vi "Check Adept Runtime.vi"(8 "Error In":errorcluster) -> (0 "Error Out":errorcluster, 2 "Installed?":bool)   [LabVIEW 2011]
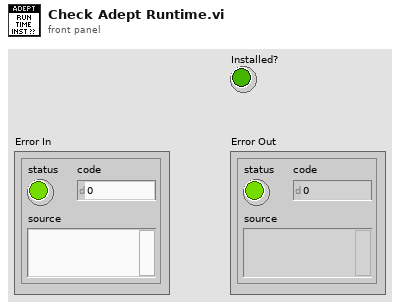
[diagram p1: front panel]
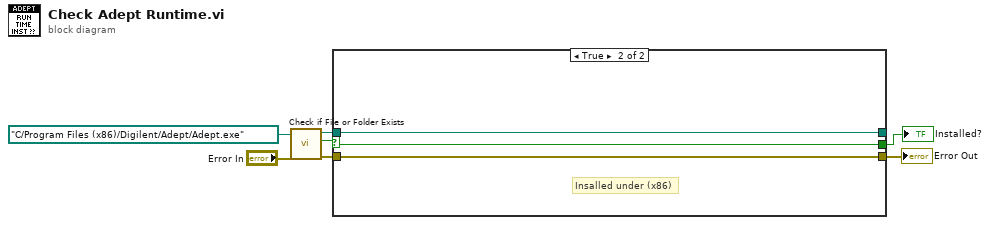
[diagram p0: block diagram]
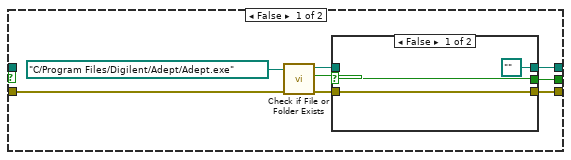
[diagram p2: hidden frame]
diagram:
  n1 = call <vilib>:"Check if File or Folder Exists.vi"("error in (no error)"="Error In", "path"=path "C:/Program Files (x86)/Digilent/Adept/Adept.exe") -> ("error out"=w4:errorcluster, "file or folder exists?"=w6:bool, "dup path"=w5:path)  [unwired: 7 in]
  n2 = case shown="True" w6 {
    selector: w6 -> [_ w22]
    tunnel: w5 -> [_ w24]
    tunnel: w4 -> [w14 w23]
    tunnel: [w13 w24] -> _
    tunnel: [w9 w23] -> w2
    tunnel: [w8 w22] -> w1
    frame False {
      n3 = call <vilib>:"Check if File or Folder Exists.vi"("error in (no error)"=w14, "path"=path "C:/Program Files/Digilent/Adept/Adept.exe") -> ("error out"=w10:errorcluster, "file or folder exists?"=w11:bool, "dup path"=w12:path)  [unwired: 7 in]
      n4 = case shown="False" w11 {
        selector: w11 -> [w17 w19]
        tunnel: [path "" ("dup path") w21] -> w13
        tunnel: w12 -> [_ w21]
        tunnel: w10 -> [w18 w20]
        tunnel: [w18 w20] -> w9
        tunnel: [w17 w19] -> w8
        frame False {
        }
        frame True {
        }
      }
    }
    frame True {
      # "Insalled under (x86)"
    }
  }
  "Error Out" <- w2
  "Installed?" <- w1
